vi "NF87XX.contents.vi"   [LabVIEW 2014, in "NF87XX.lvlib"]
uses:
  NF87XX.lvlib
panel:
  # "This is the contens.vi of the NF87XX class."
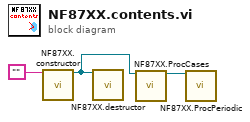
[diagram p0: block diagram]
diagram:
  n1 = call "NF87XX.constructor.vi"("name"="") -> ("i ref out"=w1:refnum<vi>)  [unwired: 16 in, 2 out]
  n2 = call "NF87XX.destructor.vi"("i ref in"=w1) -> ()  [unwired: 18 in, 1 out]
  n3 = call "NF87XX.ProcCases.vi"("i ref in"=w1) -> ("i ref out"=w3:refnum<vi>)  [unwired: 16 in, 2 out]
  n4 = call "NF87XX.ProcPeriodic.vi"("i ref in"=w3) -> ()  [unwired: 16 in, 3 out]
